vi "CreateWriteChunks.vi"(2 "chunk size (4096)":i32=4096, 3 "String":string) -> (0 "chuncks":cluster{"result string":string}[](array[cluster]))   [LabVIEW 2012]
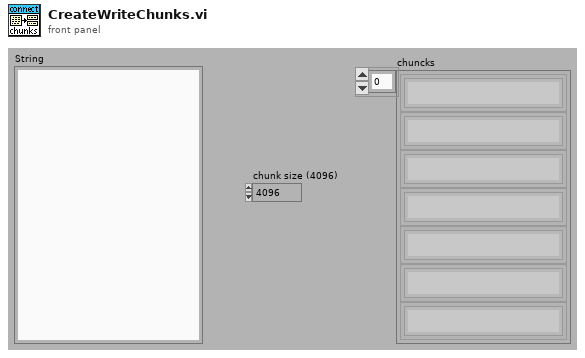
[diagram p1: front panel]
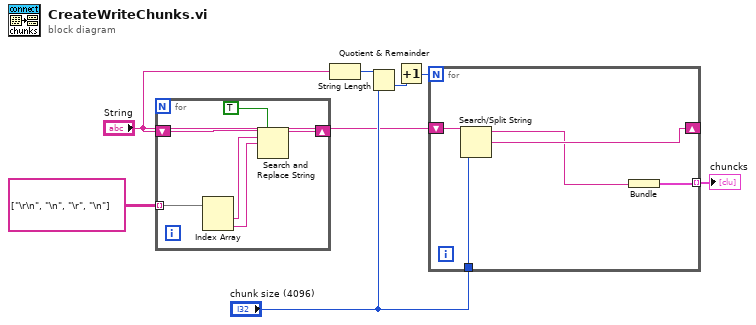
[diagram p0: block diagram]
diagram:
  n1 = for {
    tunnel: string[][] [["\r\n", "\n"], ["\r", "\n"]] -> [w13] mode=indexing
    shift-right: [w9] -> _
    shift-left: "String" -> [w12]
    n2 = Index Array(array=w13) -> (element #1=w11:string, element #2=w10:string)  [unwired: 2 in]
    n3 = Search and Replace String(replace all?=TRUE ("replace all? (F)"), input string=w12, search string=w11, replace string=w10) -> (result string=w9:string)  [unwired: 4 in, 3 out]
  }
  n4 = String Length(string="String") -> (length=w4:i32)
  n5 = Quotient & Remainder(x=w4, y="chunk size (4096)") -> (floor(x/y)=w5:i32)  [unwired: 1 out]
  n6 = Increment(x=w5) -> (x+1=w2:i32)
  n7 = for {
    N: w2 -> [_]
    shift-right: [w16] -> _
    shift-left: "String" -> [w18]
    tunnel: "chunk size (4096)" -> [w17]
    tunnel: [w15] -> w6 mode=indexing
    n8 = Search/Split String(string=w18, offset (0)=w17) -> (substring before match=w14:string, match + rest of string=w16:string)  [unwired: 2 out]
    n9 = Bundle("String"=w14) -> (w15:cluster{"String":string})  [unwired: 1 in]
  }
  "chuncks" <- w6
